vi "poly_sub_filter_multi_xwav.vi"(6 "add info? (T)":bool=TRUE, 8 "error in (no error)":errorcluster, 9 "f":i32=50 caption="base frequency (50Hz)", 10 "N":i32=3 caption="N of harmonics to remove (3)", 11 "array of xwavs in":T1) -> (0 "error out":errorcluster, 3 "array of xwavs out":T1)   [LabVIEW 2015]
uses:
  xwave/array_of_xwav.ctl
  xwave/xwav.ctl
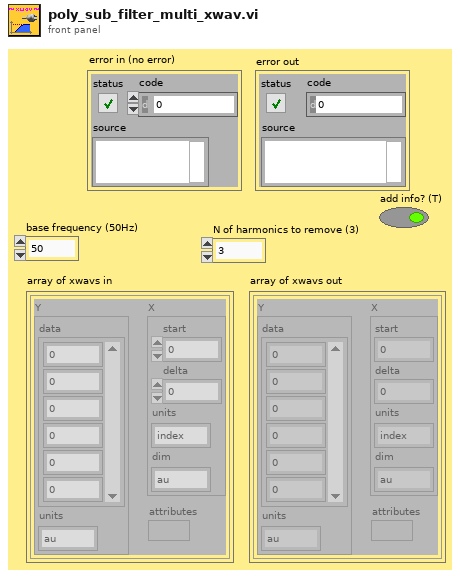
[diagram p1: front panel]
types:
  T1 = typedef "array_of_xwav.ctl" = T2[]
  T2 = typedef "xwav.ctl" = cluster{"attributes":variant, "X":cluster{"start":dbl, "delta":dbl, "units":string, "dim":string}, "Y":cluster{"data":dbl[], "units":string}}
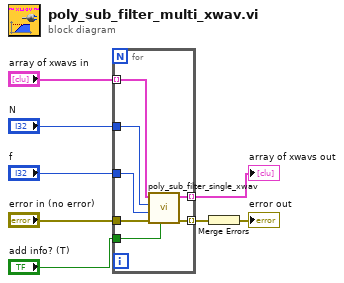
[diagram p0: block diagram]
diagram:
  n1 = for {
    tunnel: "N" -> [w15]
    tunnel: "f" -> [w14]
    tunnel: "error in (no error)" -> [w13]
    tunnel: [w12] -> w2 mode=indexing
    tunnel: [w11] -> w5 mode=indexing
    tunnel: "array of xwavs in" -> [w10] mode=indexing
    tunnel: "add info? (T)" -> [w9]
    n2 = call "poly_sub_filter_single_xwav.vi"("add info? (T)"=w9, "error in (no error)"=w13, "f"=w14, "N"=w15, "xwave in"=w10) -> ("error out"=w11:errorcluster, "xwave out"=w12:T2)  [unwired: 5 in]
  }
  "array of xwavs out" <- w2
  n3 = Merge Errors(w5) -> (→"error out":errorcluster)
